vi "TA_Plot_Spectra.vi"(0 "TA Data":T1) -> (7 "TA Spectra":cluster{"Array":dbl[], "Array 2":dbl[]}[](graph))   [LabVIEW 2025]
uses:
  TA_DATA.ctl
panel:
  out "Array":cluster{"Array":dbl[], "Array 2":dbl[]}[](array[cluster])
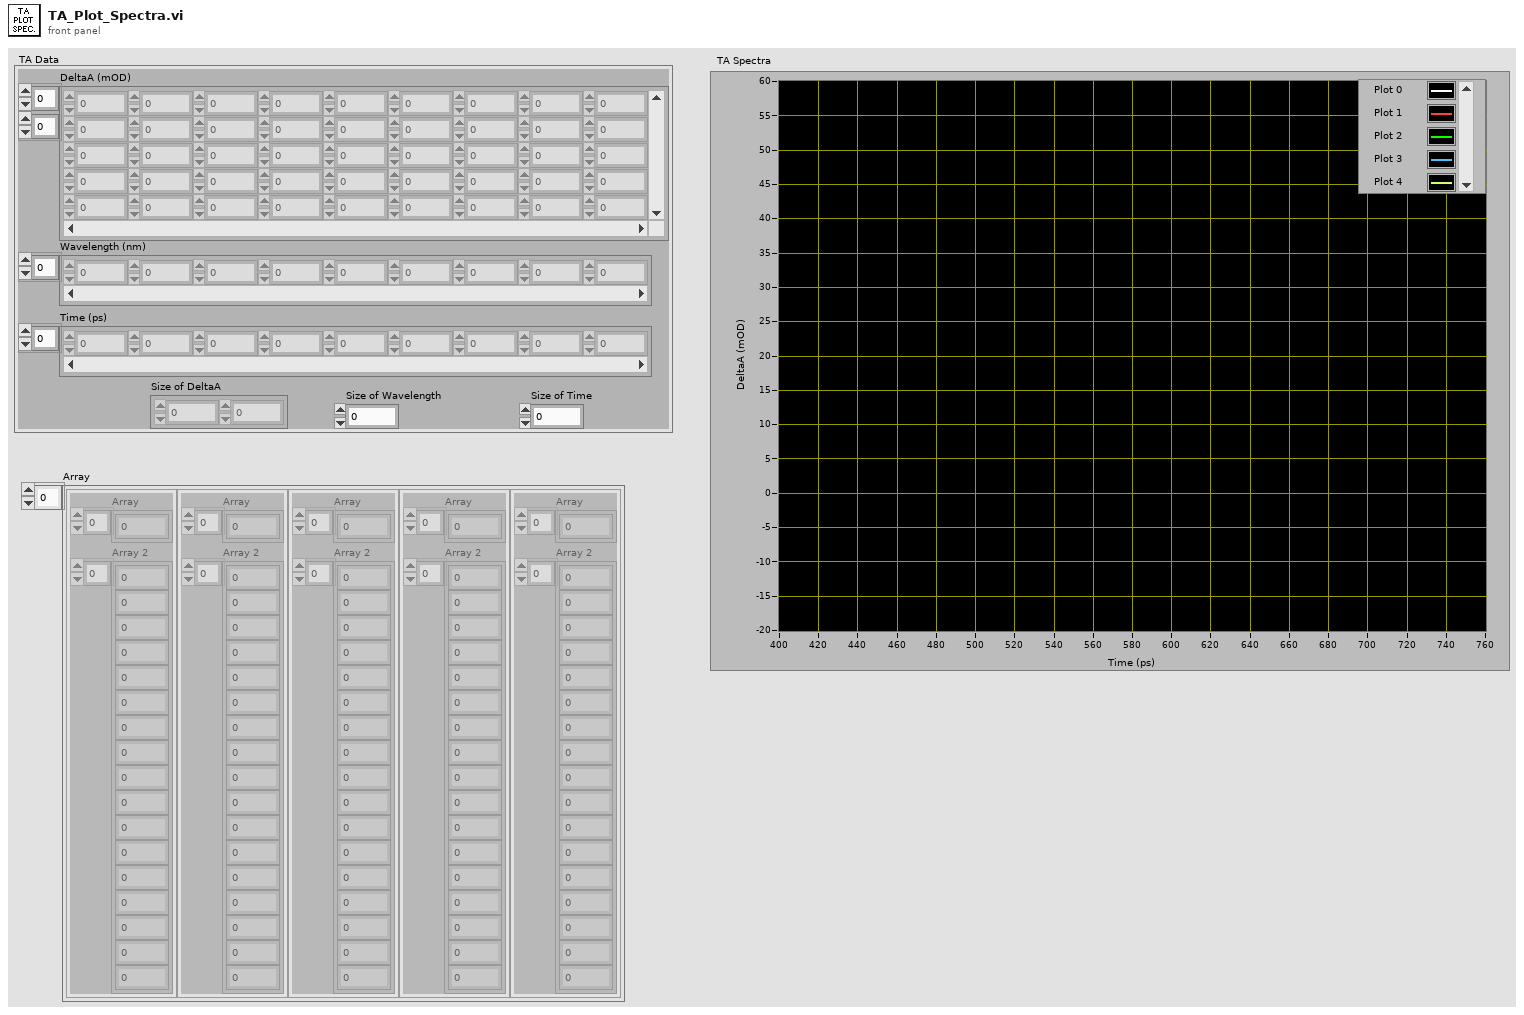
[diagram p1: front panel]
types:
  T1 = typedef "TA_DATA.ctl" = cluster{"DeltaA (mOD)":dbl[][], "Wavelength (nm)":dbl[], "Time (ps)":dbl[], "Size of DeltaA":i32[], "Size of Wavelength":i32, "Size of Time":i32}
  T2 = cluster{"Wavelength (nm)":dbl[], "DeltaA (mOD)":dbl[]}
  T3 = cluster{"Wavelength (nm)":dbl[], "DeltaA (mOD)":dbl[]}[]
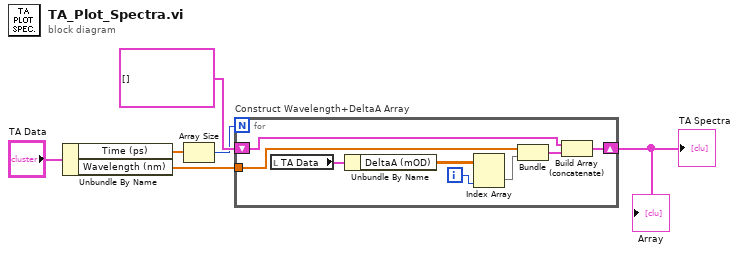
[diagram p0: block diagram]
diagram:
  n1 = Unbundle By Name("TA Data") -> ("Time (ps)"=w3:dbl[], "Wavelength (nm)"=w4:dbl[])
  n2 = Array Size(array=w3) -> (size(s)=w2:i32)
  n3 = for "Construct Wavelength+DeltaA Array" {
    N: w2 -> [_]
    tunnel: w4 -> [w14]
    shift-right: [w10] -> w6
    shift-left: cluster{"Array":dbl[], "Array 2":dbl[]}[] [] ("Array") -> [w12]
    i -> [w7]
    n4 = local read "TA Data"() -> (w9:T1)
    n5 = Unbundle By Name(w9) -> ("DeltaA (mOD)"=w8:dbl[][])
    n6 = Index Array(array=w8, index (col)=w7) -> (element=w13:dbl[])  [unwired: 1 in]
    n7 = Bundle("Wavelength (nm)"=w14, "DeltaA (mOD)"=w13) -> (w11:T2)  [unwired: 1 in]
    n8 = Build Array (concatenate)(w12, w11) -> (w10:T3)
  }
  "TA Spectra" <- w6
  "Array" <- w6
